vi "Set payload length limit.vi"(8 "error in (no error)":errorcluster, 10 "payload length limit":i32=20000, 11 "niDTS WLAN Dut in":refnum<class "niDTS WLAN Dut.lvclass">) -> (0 "error out":errorcluster, 3 "niDTS WLAN Dut out":refnum<class "niDTS WLAN Dut.lvclass">)   [LabVIEW 2015, in "niDTS WLAN.lvlib" / "niDTS WLAN Dut.lvclass"]
doc: "Sets the payload length limit. This is to ensure that payload length specifications do not exceed the capabilities of a given DUT by coercing the payload length so as not to exceed this limit.\n\nCallbacks:\n* Update Payload Length"
uses:
  niDTS WLAN Dut.lvclass
  niDTS WLAN Dut.lvclass/niDTS WLAN Dut.ctl
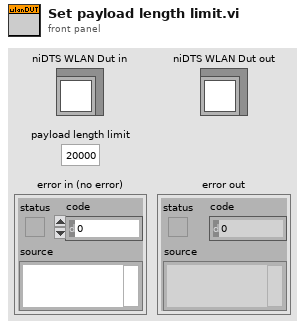
[diagram p1: front panel]
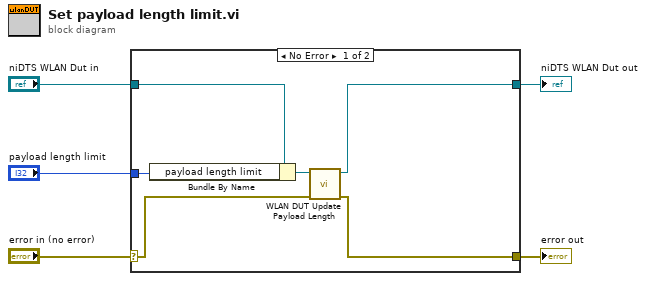
[diagram p0: block diagram]
diagram:
  n1 = case shown="No Error" "error in (no error)" {
    selector: "error in (no error)" -> [w8 w12]
    tunnel: [w7 w12] -> w4
    tunnel: [w6 w13] -> w2
    tunnel: "niDTS WLAN Dut in" -> [w11 w13]
    tunnel: "payload length limit" -> [w10 _]
    frame No Error {
      n2 = Bundle By Name(cluster=w11, "payload length limit"=w10) -> (w9:refnum<class "niDTS WLAN Dut.lvclass">)
      n3 = call-dynamic "WLAN DUT Update Payload Length.vi"("error in (no error)"=w8, "niDTS WLAN DUT in"=w9) -> ("error out"=w7:errorcluster, "niDTS WLAN DUT out"=w6:refnum<class "niDTS WLAN Dut.lvclass">)  [unwired: 8 in]
    }
    frame Error {
    }
  }
  "error out" <- w4
  "niDTS WLAN Dut out" <- w2
